vi "Store Recall Settings.vi"(8 "error in (no error)":errorcluster, 9 "location (1)":i16=1, 10 "function (T:store)":bool=TRUE, 11 "VISA resource name":refnum<visa-resource-name>) -> (0 "error out":errorcluster, 3 "VISA resource name out":refnum<visa-resource-name>)   [LabVIEW 2020, in "Agilent 6XXX Series.lvlib"]
doc: "This function allows you to store instrument setups to or recall setups from memory. This function is not supported on the HP663xA series."
uses:
  <instrlib>/Agilent 6XXX Series/Agilent 6XXX Series.lvlib
panel:
  # "HP603xA and HP662xA series only"
  # "store"
  # "recall"
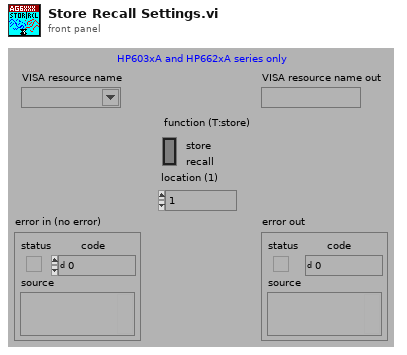
[diagram p1: front panel]
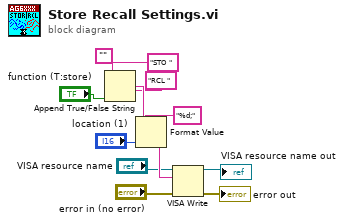
[diagram p0: block diagram]
diagram:
  n1 = Append True/False String(1:"function (T:store)", 2:"RCL ", 3:"STO ", 4:"") -> (0:w12:string)
  n2 = Format Value(string ("")=w12, format string="%d;", value (0)="location (1)") -> (output string=w5:string)
  n3 = VISA Write(VISA resource name="VISA resource name", write buffer=w5, error in (no error)="error in (no error)") -> (VISA resource name out=→"VISA resource name out":refnum<visa-resource-name>, error out=→"error out":errorcluster)  [unwired: 1 out]
